vi "HIOKI PW3390 Conf Phase Correct.vi"(0 "VISA Resource":refnum<visa-resource-name>, 1 "Set/Query (F: Set)":bool, 2 "CH (1)":i32=1 min=1 max=4, 5 "Correct (F: OFF)":bool, 7 "Frequency (kHz) (100.000)":dbl=100.0 min=0.001 max=999.999 format="%.3f", 9 "Angle (0.00)":dbl min=-90.0 max=90.0 format="%.2f", 11 "error in (no error)":errorcluster, 12 "OPC query (T: ON)":bool=TRUE, 13 "Error Out (F: Off)":bool) -> (4 "VISA Resource out":refnum<visa-resource-name>, 6 "Correct out":bool, 8 "Frequency out":dbl=100.0 format="%.3f", 10 "Angle out":dbl format="%.2f", 15 "error out":errorcluster)   [LabVIEW 2009]
doc: "Set/Query\n Set: Send the setting commands for the device.\n Query: Query the setting of the device.\n\nCorrect\n Sets phase correction formulas for current sensors.\n\nFrequency\n Sets phase correction frequency.\n Input Range: 0.001 - 999.999 (kHz)\n\nAngle\n Sets phase correction angle.\n Input Range: -90.00 - +90.00\n\n<B>Note</B>\nFrequency and Angle are valid when the Correct is ON."
panel:
  # "Note: This table may be changed by the revision. Please check the latest user manual."
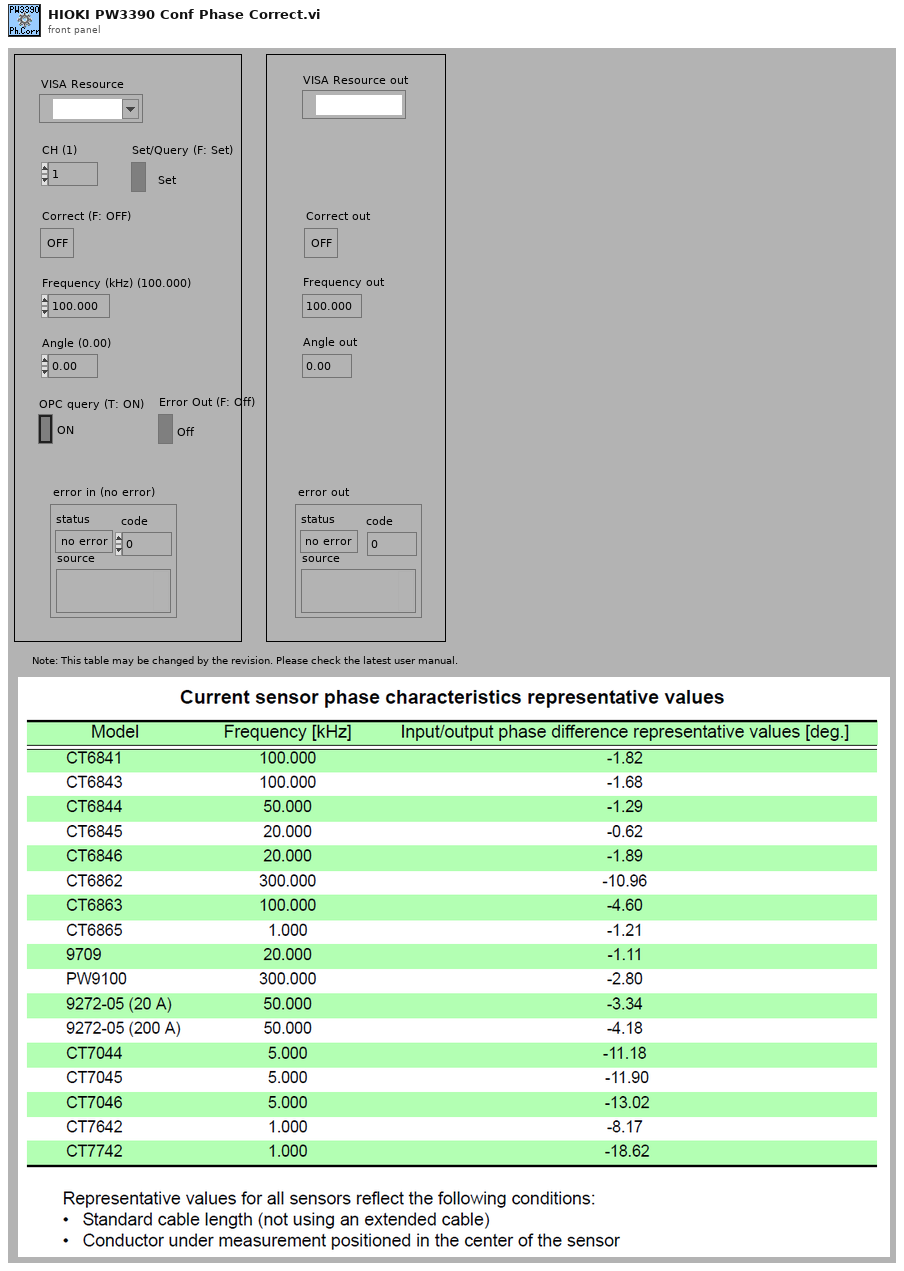
[diagram p1: front panel]
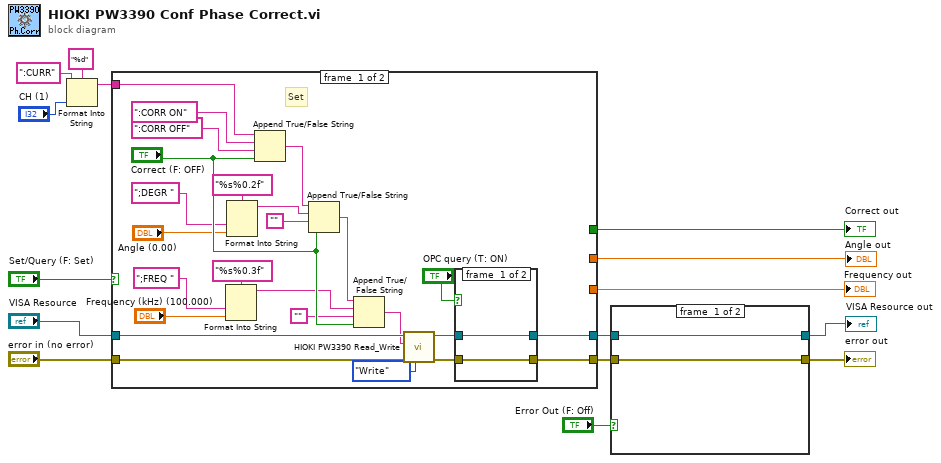
[diagram p0: block diagram]
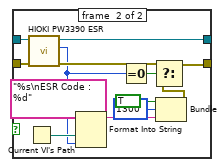
[diagram p2: hidden frame]
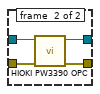
[diagram p3: hidden frame]
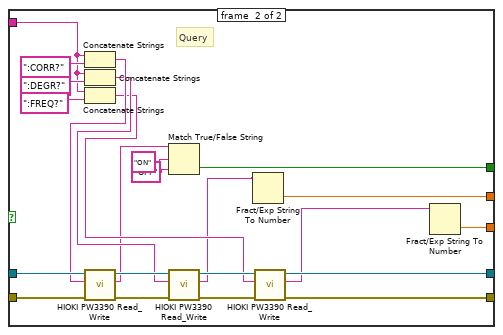
[diagram p4: hidden frame]
diagram:
  n1 = Format Into String(format string="%d", initial string=":CURR", "CH (1)") -> (resulting string=w10:string)  [unwired: 1 in, 1 out]
  n2 = case shown="FALSE" "Set/Query (F: Set)" {
    tunnel: "error in (no error)" -> [w34 w58]
    tunnel: [w27 w57] -> w8
    tunnel: "VISA Resource" -> [w35 w59]
    tunnel: [w28 w56] -> w7
    tunnel: w10 -> [w38 w66]
    tunnel: [_ w49] -> w3
    tunnel: [_ w48] -> w2
    tunnel: [_ w47] -> w1
    frame #0 {
      # "Set"
      n3 = Format Into String(format string="%s%0.3f", ";FREQ ", "Frequency (kHz) (100.000)") -> (resulting string=w21:string)  [unwired: 2 in, 1 out]
      n4 = Format Into String(format string="%s%0.2f", ";DEGR ", "Angle (0.00)") -> (resulting string=w19:string)  [unwired: 2 in, 1 out]
      n5 = Append True/False String(1:"Correct (F: OFF)", 2:":CORR OFF", 3:":CORR ON", 4:w38) -> (0:w37:string)
      n6 = Append True/False String(1:"Correct (F: OFF)", 2:"", 3:w19, 4:w37) -> (0:w36:string)
      n7 = Append True/False String(1:"Correct (F: OFF)", 2:"", 3:w21, 4:w36) -> (0:w33:string)
      n8 = call <instrlib>:"HIOKI PW3390 Read_Write.vi"("Read/Write"=enum16{"Read", "Write"}."Write", "error in (no error)"=w34, "data in"=w33, "VISA Resource"=w35) -> ("error out"=w29:errorcluster, "VISA Resource out"=w30:refnum<visa-resource-name>)  [unwired: 5 in, 1 out]
      n9 = case shown="TRUE" "OPC query (T: ON)" {
        tunnel: [w42 w46] -> w28
        tunnel: [w41 w45] -> w27
        tunnel: w30 -> [w42 w44]
        tunnel: w29 -> [w41 w43]
        frame #0 {
        }
        frame #1 {
          n10 = call <instrlib>:"HIOKI PW3390 OPC.vi"("error in (no error)"=w43, "VISA Resource"=w44) -> ("error out"=w45:errorcluster, "VISA Resource out"=w46:refnum<visa-resource-name>)  [unwired: 7 in, 1 out]
        }
      }
    }
    frame #1 {
      # "Query"
      n11 = Concatenate Strings(w66, ":CORR?") -> (w55:string)
      n12 = Concatenate Strings(w66, ":DEGR?") -> (w54:string)
      n13 = Concatenate Strings(w66, ":FREQ?") -> (w53:string)
      n14 = call <instrlib>:"HIOKI PW3390 Read_Write.vi"("error in (no error)"=w58, "data in"=w55, "VISA Resource"=w59) -> ("error out"=w62:errorcluster, "data out"=w52:string, "VISA Resource out"=w60:refnum<visa-resource-name>)  [unwired: 6 in]
      n15 = Match True/False String(2:"OFF", 3:"ON", 4:w52) -> (0:w47:bool)  [unwired: 1 out]
      n16 = call <instrlib>:"HIOKI PW3390 Read_Write.vi"("error in (no error)"=w62, "data in"=w54, "VISA Resource"=w60) -> ("error out"=w63:errorcluster, "data out"=w50:string, "VISA Resource out"=w61:refnum<visa-resource-name>)  [unwired: 6 in]
      n17 = Fract/Exp String To Number(string=w50) -> (number=w49:dbl)  [unwired: 3 in, 1 out]
      n18 = call <instrlib>:"HIOKI PW3390 Read_Write.vi"("error in (no error)"=w63, "data in"=w53, "VISA Resource"=w61) -> ("error out"=w57:errorcluster, "data out"=w51:string, "VISA Resource out"=w56:refnum<visa-resource-name>)  [unwired: 6 in]
      n19 = Fract/Exp String To Number(string=w51) -> (number=w48:dbl)  [unwired: 3 in, 1 out]
    }
  }
  "Correct out" <- w1
  "Frequency out" <- w2
  "Angle out" <- w3
  n20 = case shown="TRUE" "Error Out (F: Off)" {
    tunnel: w7 -> [w71 w84]
    tunnel: w8 -> [w70 w83]
    tunnel: [w70 w73] -> w6
    tunnel: [w71 w82] -> w4
    frame #0 {
    }
    frame #1 {
      n21 = Current VI's Path() -> (path=w80:path)
      n22 = call <instrlib>:"HIOKI PW3390 ESR.vi"("error in (no error)"=w83, "VISA Resource"=w84) -> ("error out"=w74:errorcluster, "Output Value"=w72:u8, "VISA Resource out"=w82:refnum<visa-resource-name>)  [unwired: 6 in, 1 out]
      n23 = Format Into String(format string="%s\nESR Code : %d", w80, w72) -> (resulting string=w76:string)  [unwired: 2 in, 1 out]
      n24 = Equal To 0?(x=w72) -> (x = 0?=w81:bool)
      n25 = Bundle("status"=TRUE, "code"=1300, w76) -> (w75:cluster{"status":bool, "code":i32, string})  [unwired: 1 in]
      n26 = Select(t=w74, s=w81, f=w75) -> (s? t:f=w73:errorcluster)
    }
  }
  "error out" <- w6
  "VISA Resource out" <- w4
